vi "Byte40_44 (SubVI).vi"(3 "Channel Number":dbl, 4 "Card Number":dbl, 5 "Input String 2":string) -> (1 "Cluster":T1)   [LabVIEW 2024]
panel:
  # "BYTE 43"
  # "0dan 5 e 0 =c ontrol card sw cardlarda 12345"
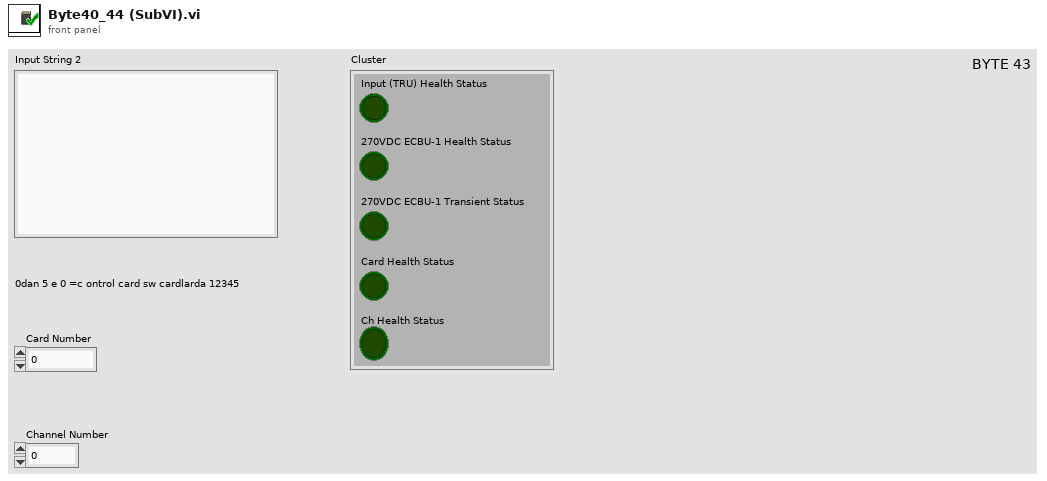
[diagram p1: front panel]
types:
  T1 = cluster{"270VDC ECBU-1 Health Status":bool, "270VDC ECBU-1 Transient Status":bool, "Input (TRU) Health Status":bool, "Card Health Status":bool, "Ch Health Status":bool}
  T2 = cluster{"Green":bool, "Gray":bool, "Yellow":bool, "White":bool, "default":bool}
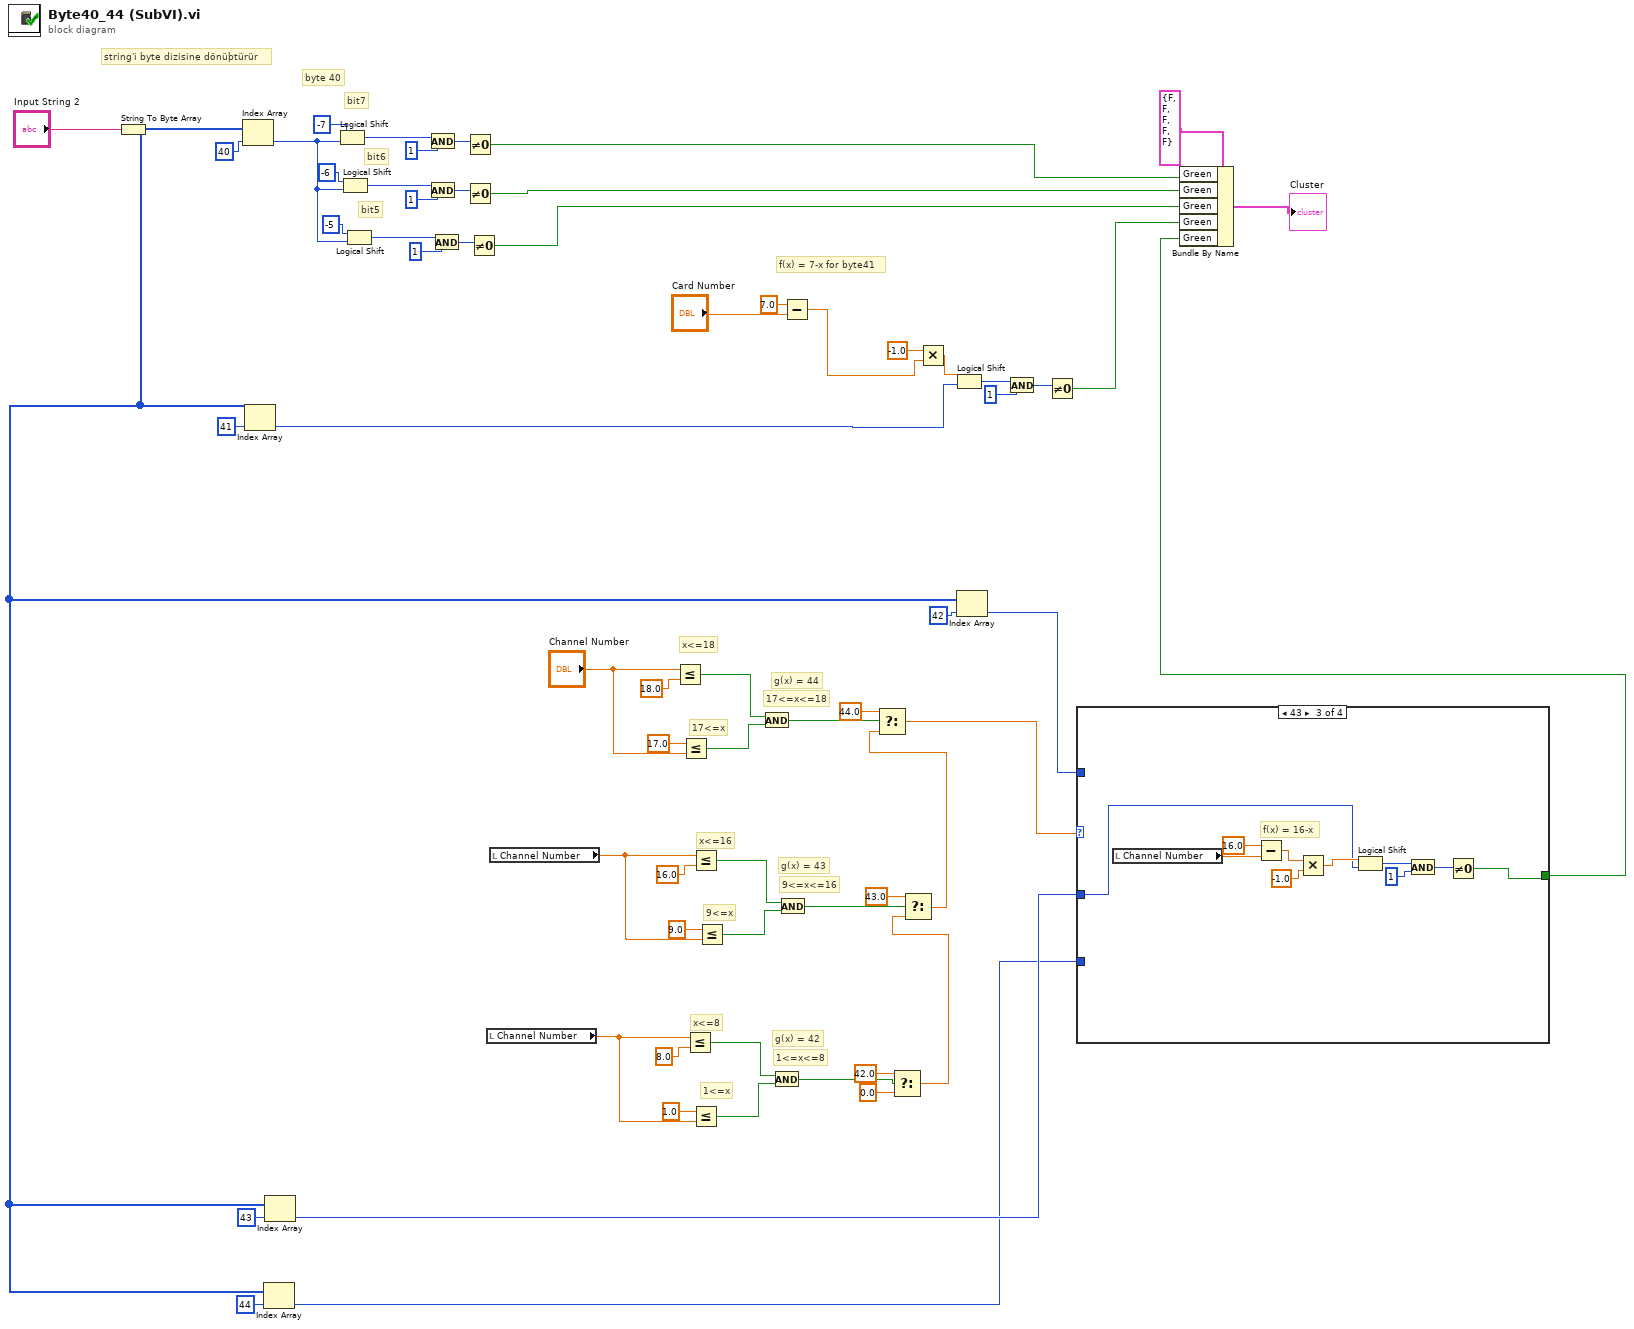
[diagram p0: block diagram]
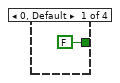
[diagram p2: hidden frame]
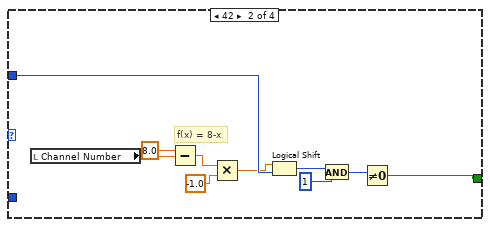
[diagram p3: hidden frame]
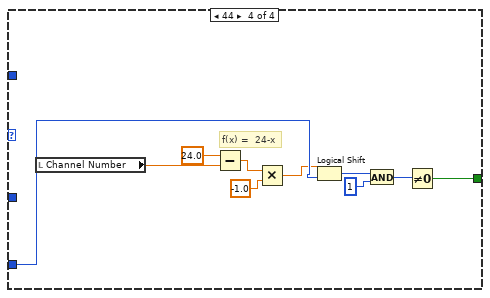
[diagram p4: hidden frame]
diagram:
  # "g(x) = 42"
  # "1<=x<=8"
  # "1<=x"
  # "x<=8"
  # "g(x) = 43"
  # "g(x) = 44"
  # "9<=x<=16"
  # "9<=x"
  # "x<=16"
  # "17<=x<=18"
  # "17<=x"
  # "x<=18"
  # "f(x) = 7-x for byte41"
  # "bit5"
  # "bit6"
  # "bit7"
  # "byte 40"
  # "string'i byte dizisine dönüþtürür"
  n1 = String To Byte Array(string="Input String 2") -> (unsigned byte array=w16:u8[])
  n2 = Index Array "Index Array"(array=w16, index=40) -> (element=w51:u8)
  n3 = Index Array(array=w16, index=41) -> (element=w8:u8)
  n4 = Index Array(array=w16, index=44) -> (element=w15:u8)
  n5 = Index Array(array=w16, index=43) -> (element=w18:u8)
  n6 = Logical Shift(y=i16 -7, x=w51) -> (x << y=w60:u8)
  n7 = Logical Shift(y=i16 -6, x=w51) -> (x << y=w56:u8)
  n8 = Logical Shift(y=i16 -5, x=w51) -> (x << y=w55:u8)
  n9 = And(x=w60, y=u8 1) -> (x .and. y?=w62:u8)
  n10 = And(x=w56, y=u8 1) -> (x .and. y?=w57:u8)
  n11 = And(x=w55, y=u8 1) -> (x .and. y?=w54:u8)
  n12 = Not Equal To 0?(x=w62) -> (x != 0?=w7:bool)
  n13 = Not Equal To 0?(x=w57) -> (x != 0?=w6:bool)
  n14 = Not Equal To 0?(x=w54) -> (x != 0?=w5:bool)
  n15 = local read "Channel Number"() -> (w30:dbl)
  n16 = local read "Channel Number"() -> (w32:dbl)
  n17 = Less Or Equal?(x="Channel Number", y=18.0) -> (x <= y?=w44:bool)
  n18 = Less Or Equal?(x=17.0, y="Channel Number") -> (x <= y?=w43:bool)
  n19 = Less Or Equal?(x=w30, y=8.0) -> (x <= y?=w36:bool)
  n20 = Less Or Equal?(x=w32, y=16.0) -> (x <= y?=w40:bool)
  n21 = Less Or Equal?(x=1.0, y=w30) -> (x <= y?=w35:bool)
  n22 = Less Or Equal?(x=9.0, y=w32) -> (x <= y?=w39:bool)
  n23 = And(x=w44, y=w43) -> (x .and. y?=w33:bool)
  n24 = And(x=w36, y=w35) -> (x .and. y?=w28:bool)
  n25 = And(x=w40, y=w39) -> (x .and. y?=w31:bool)
  n26 = Subtract(x=7.0, y="Card Number") -> (x-y=w9:dbl)
  n27 = Select(t=42.0, s=w28, f=0.0) -> (s? t:f=w22:dbl)
  n28 = Select(t=43.0, s=w31, f=w22) -> (s? t:f=w23:dbl)
  n29 = Select(t=44.0, s=w33, f=w23) -> (s? t:f=w21:dbl)
  n30 = Multiply(x=-1.0, y=w9) -> (x*y=w10:dbl)
  n31 = Logical Shift(y=w10, x=w8) -> (x << y=w13:u8)
  n32 = Index Array(array=w16, index=42) -> (element=w20:u8)
  n33 = And(x=w13, y=u8 1) -> (x .and. y?=w12:u8)
  n34 = Not Equal To 0?(x=w12) -> (x != 0?=w4:bool)
  n35 = case shown="43" w21 {
    tunnel: w20 -> [_ w67 _ _]
    tunnel: [FALSE w68 w78 w88] -> w3
    tunnel: w18 -> [_ _ w76 _]
    tunnel: w15 -> [_ _ _ w87]
    frame 0, Default {
    }
    frame 42 {
      # "f(x) = 8-x"
      n36 = local read "Channel Number"() -> (w75:dbl)
      n37 = Subtract(x=8.0, y=w75) -> (x-y=w73:dbl)
      n38 = Multiply(x=w73, y=-1.0) -> (x*y=w66:dbl)
      n39 = Logical Shift(y=w66, x=w67) -> (x << y=w70:u8)
      n40 = And(x=w70, y=u8 1) -> (x .and. y?=w69:u8)
      n41 = Not Equal To 0?(x=w69) -> (x != 0?=w68:bool)
    }
    frame 43 {
      # "f(x) = 16-x"
      n42 = local read "Channel Number"() -> (w79:dbl)
      n43 = Subtract(x=16.0, y=w79) -> (x-y=w83:dbl)
      n44 = Multiply(x=w83, y=-1.0) -> (x*y=w77:dbl)
      n45 = Logical Shift(y=w77, x=w76) -> (x << y=w84:u8)
      n46 = And(x=w84, y=u8 1) -> (x .and. y?=w85:u8)
      n47 = Not Equal To 0?(x=w85) -> (x != 0?=w78:bool)
    }
    frame 44 {
      # "f(x) =  24-x"
      n48 = local read "Channel Number"() -> (w89:dbl)
      n49 = Subtract(x=24.0, y=w89) -> (x-y=w93:dbl)
      n50 = Multiply(x=w93, y=-1.0) -> (x*y=w86:dbl)
      n51 = Logical Shift(y=w86, x=w87) -> (x << y=w94:u8)
      n52 = And(x=w94, y=u8 1) -> (x .and. y?=w95:u8)
      n53 = Not Equal To 0?(x=w95) -> (x != 0?=w88:bool)
    }
  }
  n54 = Bundle By Name "Bundle By Name"(cluster=T2 {"Green"=FALSE, "Gray"=FALSE, "Yellow"=FALSE, "White"=FALSE, "default"=FALSE} ("Ch1 Frame Color"), "Green"=w7, "Green"=w6, "Green"=w5, "Green"=w4, "Green"=w3) -> (→"Cluster":T2)
